vi "_checkW&R_EEPROM_vna_wmg.vi"(3 "EEPROMCheck":string[][](array[string])=[["0", "1", "0", "3"], ["0", "1", "10", "14"], ["0", "3", "2", "4"]], 4 "ref_read_ports":refnum<vi>[](array[refnum]), 5 "ref_temp_ports":refnum<vi>[](array[refnum]), 6 "portNum":i32) -> (0 "mes":string, 1 "result_A":bool[](array[boolean]), 2 "result":bool)   [LabVIEW 2011]
panel:
  out "数值":i32
  out "值 2":string[][](array[string])
  out "值":string[][](array[string])
  out "r_ports":bool[](array[boolean])
  out "message_1":string
  out "message":string
  # "格式为\nport          col           startbyte    endbyte\n端口号       列数          起始字节      结束字节"
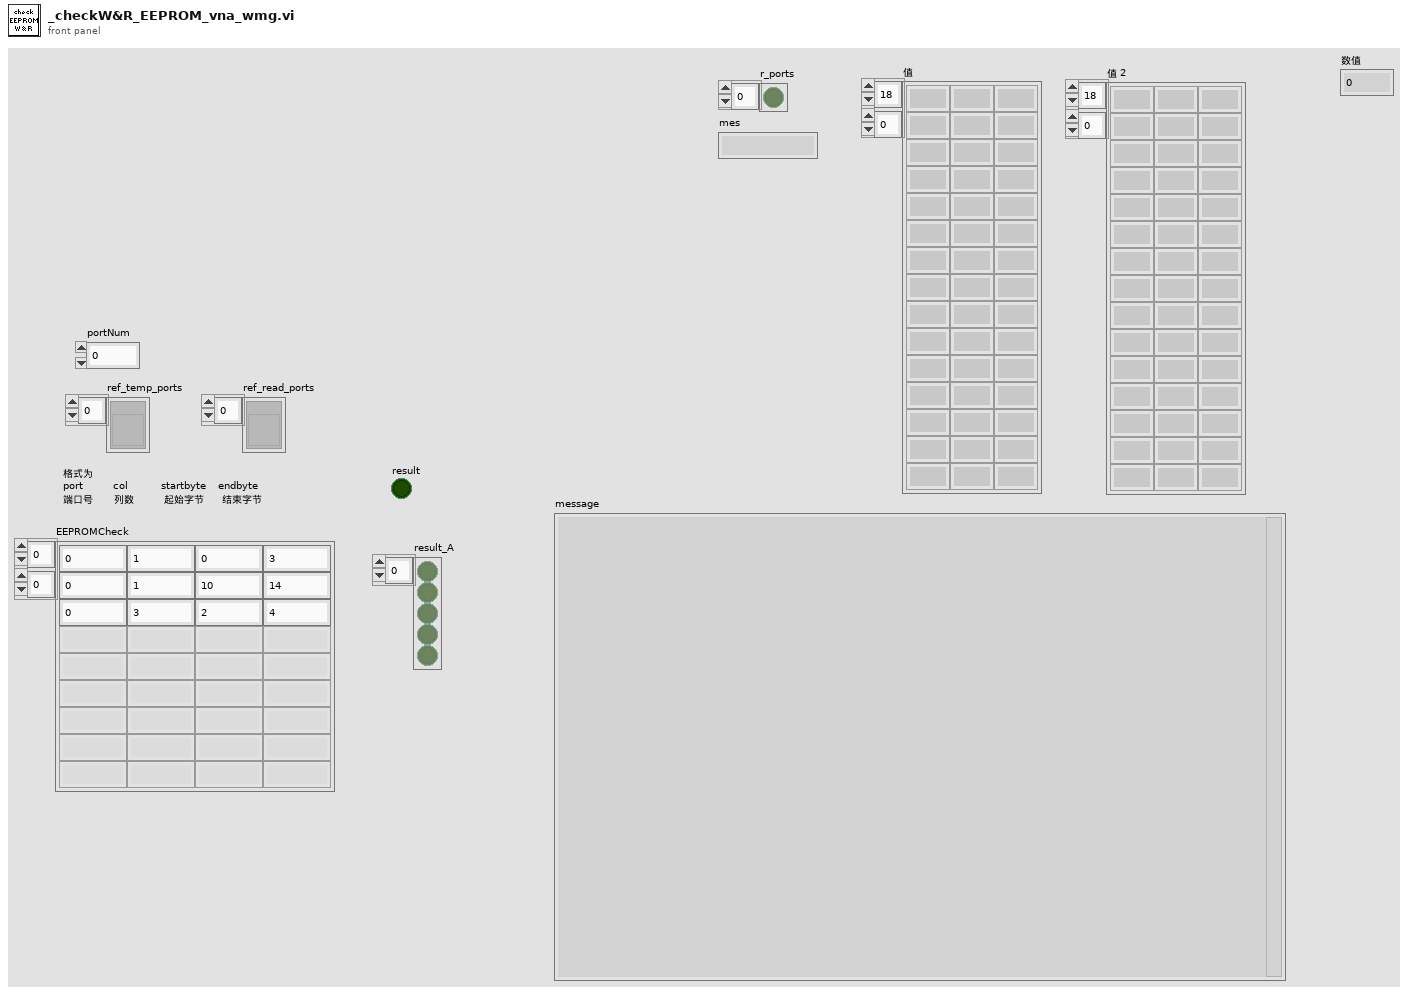
[diagram p1: front panel]
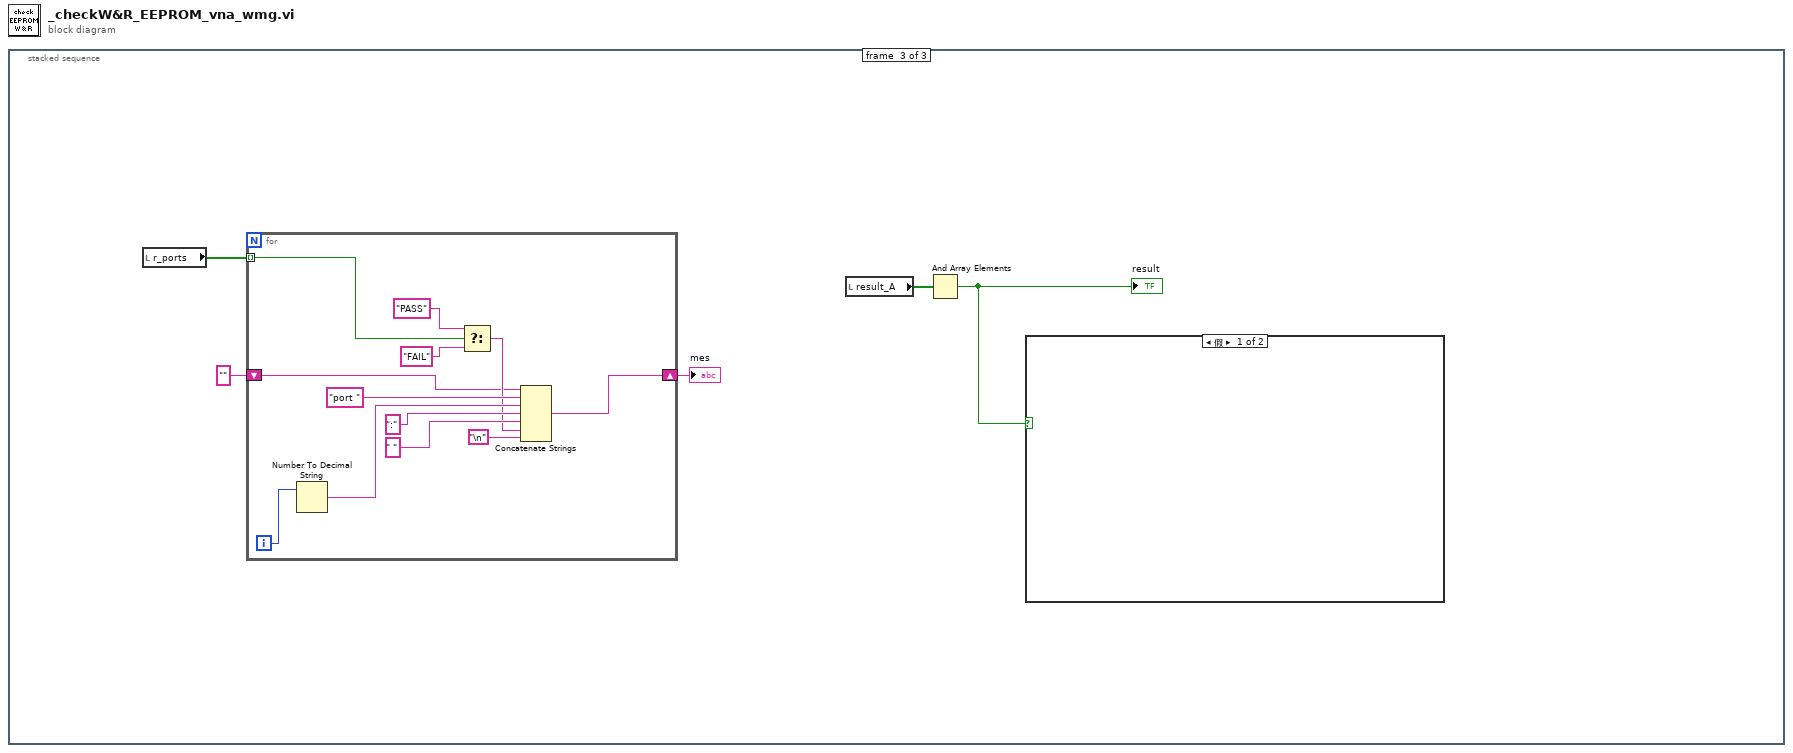
[diagram p0: block diagram]
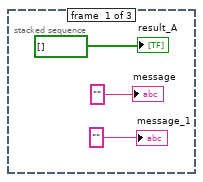
[diagram p2: hidden frame]
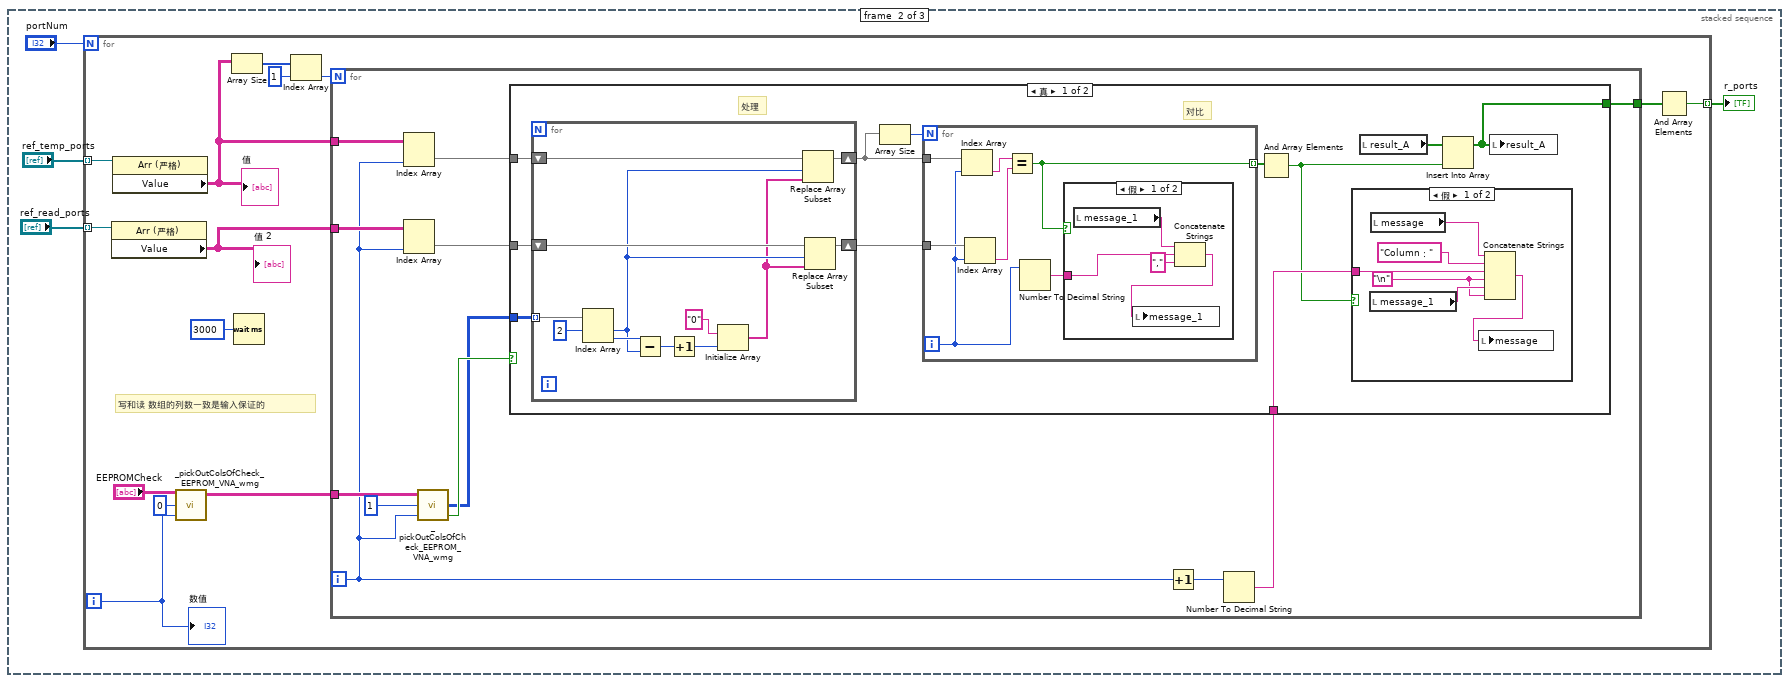
[diagram p3: hidden frame]
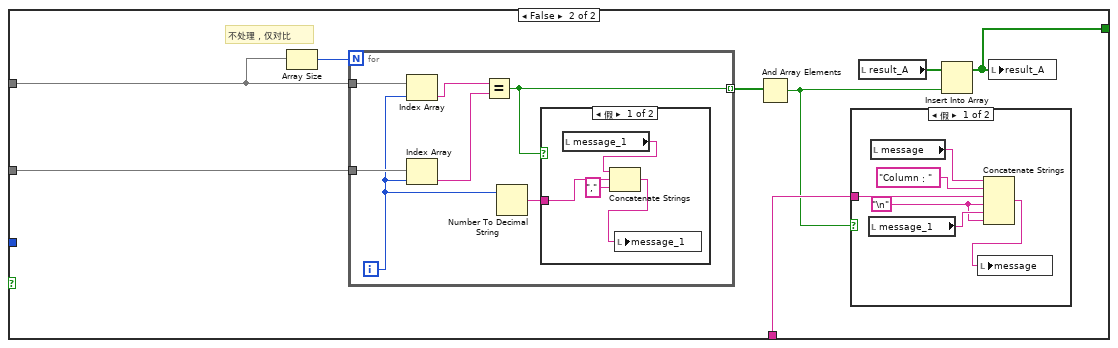
[diagram p6: hidden frame]
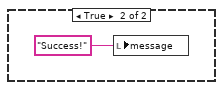
[diagram p9: hidden frame]
diagram:
  n1 = stacked-sequence {
    frame #0 {
      "result_A" <- bool[] []
      "message" <- ""
      "message_1" <- "" ("message_1")
    }
    frame #1 {
      n2 = for {
        N: "portNum" -> [_]
        tunnel: "ref_temp_ports" -> [w18] mode=indexing
        tunnel: "ref_read_ports" -> [w16] mode=indexing
        tunnel: [w9] -> w4 mode=indexing
        i -> [w12]
        # "写和读 数组的列数一致是输入保证的"
        n3 = property class="Arr (严格)"(reference=w16) -> ("Value"=w15:string[][])  [unwired: 1 in, 2 out]
        "值 2" <- w15
        n4 = property class="Arr (严格)"(reference=w18) -> ("Value"=w17:string[][])  [unwired: 1 in, 2 out]
        "值" <- w17
        n5 = call "_pickOutColsOfCheck_EEPROM_VNA_wmg.vi"("sys_index"=w12, "indexToBeFind"=0, "EEPROMCheck"="EEPROMCheck") -> ("output"=w11:string[][])  [unwired: 2 out]
        n6 = Array Size(array=w17) -> (size(s)=w21:i32[])
        n7 = Wait (ms)(milliseconds to wait=u32 3000 ("等待时间（毫秒）")) -> ()  [unwired: 1 out]
        n8 = Index Array(array=w21, index=1 ("索引")) -> (element=w19:i32)
        n9 = for {
          N: w19 -> [_]
          tunnel: w17 -> [w33]
          tunnel: w15 -> [w32]
          tunnel: w11 -> [w27]
          tunnel: [w22] -> w10
          i -> [w25]
          n10 = Index Array(array=w33, index (col)=w25) -> (element=w31:string[])  [unwired: 1 in]
          n11 = Index Array(array=w32, index (col)=w25) -> (element=w30:string[])  [unwired: 1 in]
          n12 = call "_pickOutColsOfCheck_EEPROM_VNA_wmg.vi"("sys_index"=w25, "indexToBeFind"=1, "EEPROMCheck"=w27) -> ("x != y?"=w24:bool, "output"=w23:i32[][])  [unwired: 1 out]
          n13 = Increment(x=w25) -> (x+1=w28:i32)
          n14 = Number To Decimal String(number=w28) -> (decimal integer string=w29:string)  [unwired: 1 in]
          n15 = case shown="真" w24 {
            tunnel: w23 -> [w44 _]
            tunnel: w31 -> [w43 w74]
            tunnel: w30 -> [w42 w77]
            tunnel: w29 -> [w39 w80]
            tunnel: [w36 w76] -> w22
            frame True {
              # "处理"
              # "对比"
              n16 = for {
                tunnel: w44 -> [w73] mode=indexing
                shift-right: [w63] -> w34
                shift-left: w43 -> [w71]
                shift-right: [w62] -> w41
                shift-left: w42 -> [w66]
                n17 = Index Array(array=w73, index #1=2 ("索引")) -> (element #1=w65:i32, element #2=w70:i32)  [unwired: 1 in]
                n18 = Subtract(x=w70, y=w65) -> (x-y=w69:i32)
                n19 = Increment(x=w69) -> (x+1=w68:i32)
                n20 = Initialize Array("0", w68) -> (w64:string[])
                n21 = Replace Array Subset(array=w71, new element=w64, index=w65) -> (w63:string[])
                n22 = Replace Array Subset(array=w66, new element=w64, index=w65) -> (w62:string[])
              }
              n23 = Array Size(array=w34) -> (size(s)=w35:i32)
              n24 = for {
                N: w35 -> [_]
                tunnel: w34 -> [w55]
                tunnel: w41 -> [w53]
                tunnel: [w57] -> w40 mode=indexing
                i -> [w52]
                n25 = Index Array(array=w55, index=w52) -> (element=w54:string)
                n26 = Index Array(array=w53, index=w52) -> (element=w51:string)
                n27 = Equal?(x=w54, y=w51) -> (x = y?=w57:bool)
                n28 = Number To Decimal String(number=w52) -> (decimal integer string=w56:string)  [unwired: 1 in]
                n29 = case shown="假" w57 {
                  tunnel: w56 -> [w60 _]
                  frame False {
                    n30 = local read "message_1"() -> (w61:string)
                    n31 = Concatenate Strings(w61, w60, "," ("字符串")) -> (w58:string)
                    n32 = local write "message_1"(w58) -> ()
                  }
                  frame True {
                  }
                }
              }
              n33 = And Array Elements(Boolean array=w40) -> (logical AND=w37:bool)
              n34 = case shown="假" w37 {
                tunnel: w39 -> [w50 _]
                frame False {
                  w48 = "\n"
                  n35 = local read "message_1"() -> (w49:string)
                  n36 = local read "message"() -> (w45:string)
                  n37 = Concatenate Strings(w45, "Column：", w50, w48, w49, w48) -> (w47:string)
                  n38 = local write "message"(w47) -> ()
                }
                frame True {
                }
              }
              n39 = local read "result_A"() -> (w38:bool[])
              n40 = Insert Into Array(array=w38, new element=w37) -> (w36:bool[])  [unwired: 1 in]
              n41 = local write "result_A"(w36) -> ()
            }
            frame False {
              # "不处理，仅对比"
              n42 = Array Size(array=w74) -> (size(s)=w75:i32)
              n43 = for {
                N: w75 -> [_]
                tunnel: w74 -> [w92]
                tunnel: w77 -> [w90]
                tunnel: [w94] -> w81 mode=indexing
                i -> [w89]
                n44 = Index Array(array=w92, index=w89) -> (element=w91:string)
                n45 = Index Array(array=w90, index=w89) -> (element=w88:string)
                n46 = Equal?(x=w91, y=w88) -> (x = y?=w94:bool)
                n47 = Number To Decimal String(number=w89) -> (decimal integer string=w93:string)  [unwired: 1 in]
                n48 = case shown="假" w94 {
                  tunnel: w93 -> [w98 _]
                  frame False {
                    n49 = local read "message_1"() -> (w95:string)
                    n50 = Concatenate Strings(w95, w98, "," ("字符串")) -> (w96:string)
                    n51 = local write "message_1"(w96) -> ()
                  }
                  frame True {
                  }
                }
              }
              n52 = And Array Elements(Boolean array=w81) -> (logical AND=w78:bool)
              n53 = case shown="假" w78 {
                tunnel: w80 -> [w86 _]
                frame False {
                  w84 = "\n"
                  n54 = local read "message_1"() -> (w85:string)
                  n55 = local read "message"() -> (w82:string)
                  n56 = Concatenate Strings(w82, "Column：", w86, w84, w85, w84) -> (w83:string)
                  n57 = local write "message"(w83) -> ()
                }
                frame True {
                }
              }
              n58 = local read "result_A"() -> (w79:bool[])
              n59 = Insert Into Array(array=w79, new element=w78) -> (w76:bool[])  [unwired: 1 in]
              n60 = local write "result_A"(w76) -> ()
            }
          }
        }
        n61 = And Array Elements(Boolean array=w10) -> (logical AND=w9:bool)
        "数值" <- w12
      }
      "r_ports" <- w4
    }
    frame #2 {
      n62 = local read "r_ports"() -> (w101:bool[])
      n63 = for {
        tunnel: w101 -> [w108] mode=indexing
        shift-right: [w105] -> w99
        shift-left: "" -> [w104]
        i -> [w115]
        n64 = Number To Decimal String(number=w115) -> (decimal integer string=w113:string)  [unwired: 1 in]
        n65 = Select(t="PASS", s=w108, f="FAIL") -> (s? t:f=w107:string)
        n66 = Concatenate Strings(w104, "port ", w113, ":", " ", w107, "\n") -> (w105:string)
      }
      "mes" <- w99
      n67 = local read "result_A"() -> (w103:bool[])
      n68 = And Array Elements(Boolean array=w103) -> (logical AND=w102:bool)
      "result" <- w102
      n69 = case shown="假" w102 {
        frame False {
        }
        frame True {
          n70 = local write "message"("Success!" ("message")) -> ()
        }
      }
    }
  }
